vi "Get and Set RT Menu Path.vi"(8 "错误输入（无错误）":errorcluster, 10 "RT Menu Path In":path, 11 "VI Ref In":refnum<vi>) -> (0 "错误输出":errorcluster, 2 "RT Menu Path out":path, 3 "VI Ref Out":refnum<vi>)   [LabVIEW 2012, in "VIRef.lvlib"]
uses:
  VIRef.lvlib
panel:
  in  "Mode":enum16{"Read", "Write"}(ring)
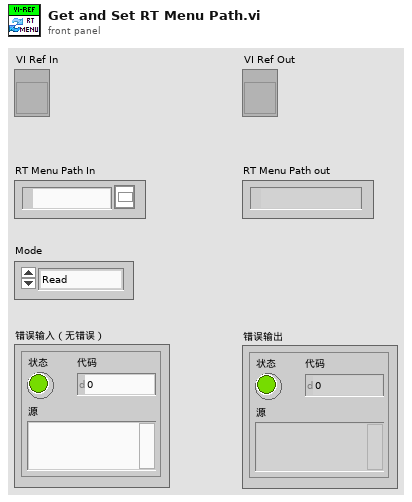
[diagram p1: front panel]
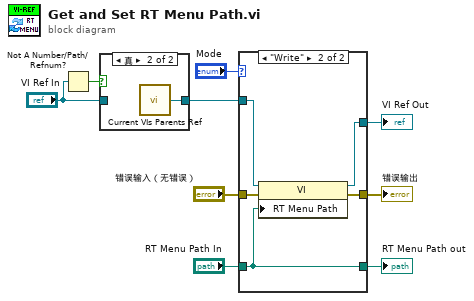
[diagram p0: block diagram]
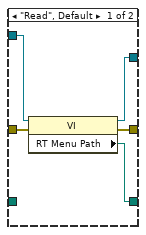
[diagram p2: hidden frame]
diagram:
  n1 = Not A Number/Path/Refnum?(number/path/refnum="VI Ref In") -> (NaN/Path/Refnum?=w9:bool)
  n2 = case shown="真" w9 {
    tunnel: [w10 w11] -> w4
    tunnel: "VI Ref In" -> [w10 _]
    frame False {
    }
    frame True {
      n3 = call "Current VIs Parents Ref.vi"() -> ("Calling VI's Reference"=w11:refnum<vi>)  [unwired: 2 in]
    }
  }
  n4 = case shown="\"Write\"" "Mode" {
    tunnel: "错误输入（无错误）" -> [w16 w21]
    tunnel: [w15 w20] -> w5
    tunnel: w4 -> [w14 w19]
    tunnel: [w13 w18] -> w3
    tunnel: "RT Menu Path In" -> [_ w17]
    tunnel: [w12 w17] -> w1
    frame "Read", Default {
      n5 = property class="VI"(reference=w14, error in=w16) -> (reference out=w13:refnum<vi>, error out=w15:errorcluster, "RT Menu Path"=w12:path)
    }
    frame "Write" {
      n6 = property class="VI"(reference=w19, error in=w21, "RT Menu Path"=w17) -> (reference out=w18:refnum<vi>, error out=w20:errorcluster)
    }
  }
  "错误输出" <- w5
  "VI Ref Out" <- w3
  "RT Menu Path out" <- w1
